vi "Elevator Controller.vi"(8 "error in":errorcluster) -> ()   [LabVIEW 2018]
doc: "This VI executes continuously carrying out the current operation and responding to updates or new operations. It will often contain the timing or control code that is difficult to place directly in TeleOp. This VI generally opens all sensors and motors and isolates the rest of the robot code from knowing how the operations are carried out."
uses:
  <vilib>/Rock Robotics/WPI/Framework/Completion Status.ctl
  Elevator Setpoints.ctl
  Elevator Operations.ctl
  <vilib>/Rock Robotics/WPI/SafetyOutput/WPI_SafetyOutputConfigMenu.ctl
  <vilib>/Rock Robotics/WPI/Utilities/WPI_GetSetVariantRefNum.vi
  <vilib>/Rock Robotics/Network Tables/NT Write Boolean.vi
panel:
  in  "Interactive Values":T1
  out "Current\nCmd":string
  in  "Buttons":cluster{"Execute Cmd":bool, "Abort Cmd":bool}
  out "Command Timing":cluster{"Start Time (ms)":u32, "Iterations":i32}
  out "Status":T3
  # "Tip: It may be helpful to observe inputs and sensor values.\nYou may also want to display tuning or debugging controls."
  # "Interactive Command: You may fill in the settings for a command\nand schedule it with the Execute button. You can observe and abort\nany command while fine tuning the code for the controller."
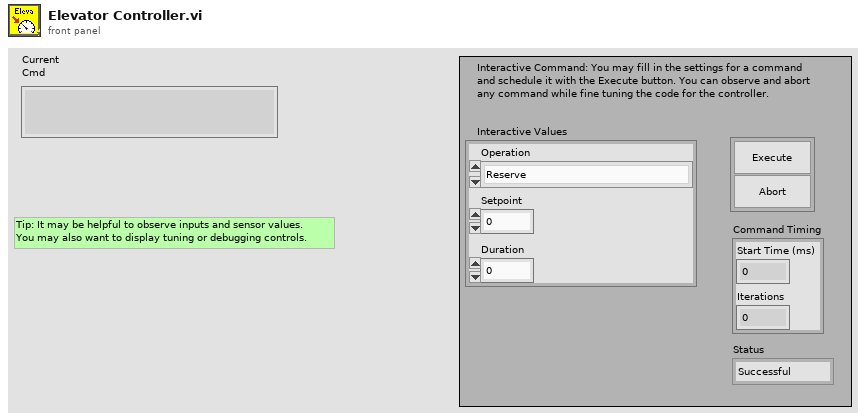
[diagram p1: front panel]
types:
  T1 = typedef "Elevator Setpoints.ctl" = cluster{"Operation":T2, "Setpoint":dbl, "Duration":dbl}
  T2 = typedef "Elevator Operations.ctl" = enum16{"Reserve", "Read Current", "Immediate"}
  T3 = typedef "Completion Status.ctl" = enum16{"Successful", "Aborted", "Incomplete"}
  T4 = typedef "WPI_SafetyOutputConfigMenu.ctl" = enum16{"Enable", "Disable"}
  T5 = typedef "WPI_RobotDriveDevRef.ctl" = cluster{"DevStatus":errorcluster, "Motors[]":T6[], "Square Inputs":bool, "Max Output":dbl}
  T6 = typedef "WPI_MotorControlDeviceRef.ctl" = cluster{"DeviceStatus":errorcluster, "Type":T7, "PWM":cluster{"PWM Channel":T8, "DeadBand":T9}, "CAN":cluster{"Device Number":u8, "SetOutput VI Ref":variant, "GetOutput VI Ref":variant, "Enable VI Ref":variant, "Disable VI Ref":variant, "Data":variant}, "Invert":bool, "DIO PWM":cluster{"PWM \"Enable\" Channel":T8, "DIOChannel":T10, "PWM Rate":dbl}}
  T7 = typedef "WPI_MotorControlType.ctl" = enum16{"PWM", "CAN", "DIO PWM"}
  T8 = typedef "FPGA_DIOPWMChannel.ctl" = enum8{"PWM 0", "PWM 1", "PWM 2", "PWM 3", "PWM 4", "PWM 5", "PWM 6", "PWM 7", "PWM 8", "PWM 9", "PWM MXP 0", "PWM MXP 1", "PWM MXP 2", "PWM MXP 3", "PWM MXP 4", "PWM MXP 5", "PWM MXP 6", "PWM MXP 7", "PWM MXP 8", "PWM MXP 9", "Invalid"}
  T9 = typedef "WPI_PWMDeadband.ctl" = cluster{"Name":string, "maxPositivePwm":i32, "minPositivePwm":i32, "centerPwm":i32, "maxNegativePwm":i32, "minNegativePwm":i32, "angularRange":u16}
  T10 = typedef "FPGA_DIOChannel.ctl" = enum8{"DIO 0", "DIO 1", "DIO 2", "DIO 3", "DIO 4", "DIO 5", "DIO 6", "DIO 7", "DIO 8", "DIO 9", "DIO MXP 0", "DIO MXP 1", "DIO MXP 2", "DIO MXP 3", "DIO MXP 4", "DIO MXP 5", "DIO MXP 6", "DIO MXP 7", "DIO MXP 8", "DIO MXP 9", "DIO MXP 10", "DIO MXP 11", "DIO MXP 12", "DIO MXP 13", "DIO MXP 14", "DIO MXP 15", "SPI Port CS1", "SPI Port CS2", "SPI Port CS3", "SPI Port MISO", "SPI Port MOSI", "Invalid"}
  T11 = typedef "Command Status Info.ctl" = cluster{"Name":string, "Status":T3, "notifier out":T12}
  T12 = typedef "Completion Notifier.ctl" = refnum<notifier>
  T13 = cluster{"Current Command":T1, "Command Timing":cluster{"Start Time (ms)":u32, "Iterations":i32}, "Command Arguments":cluster{"Command Info":T11, "Description":string, "Default Command":T1, "queue out":refnum<queue>, "Subsystem Name":string}}
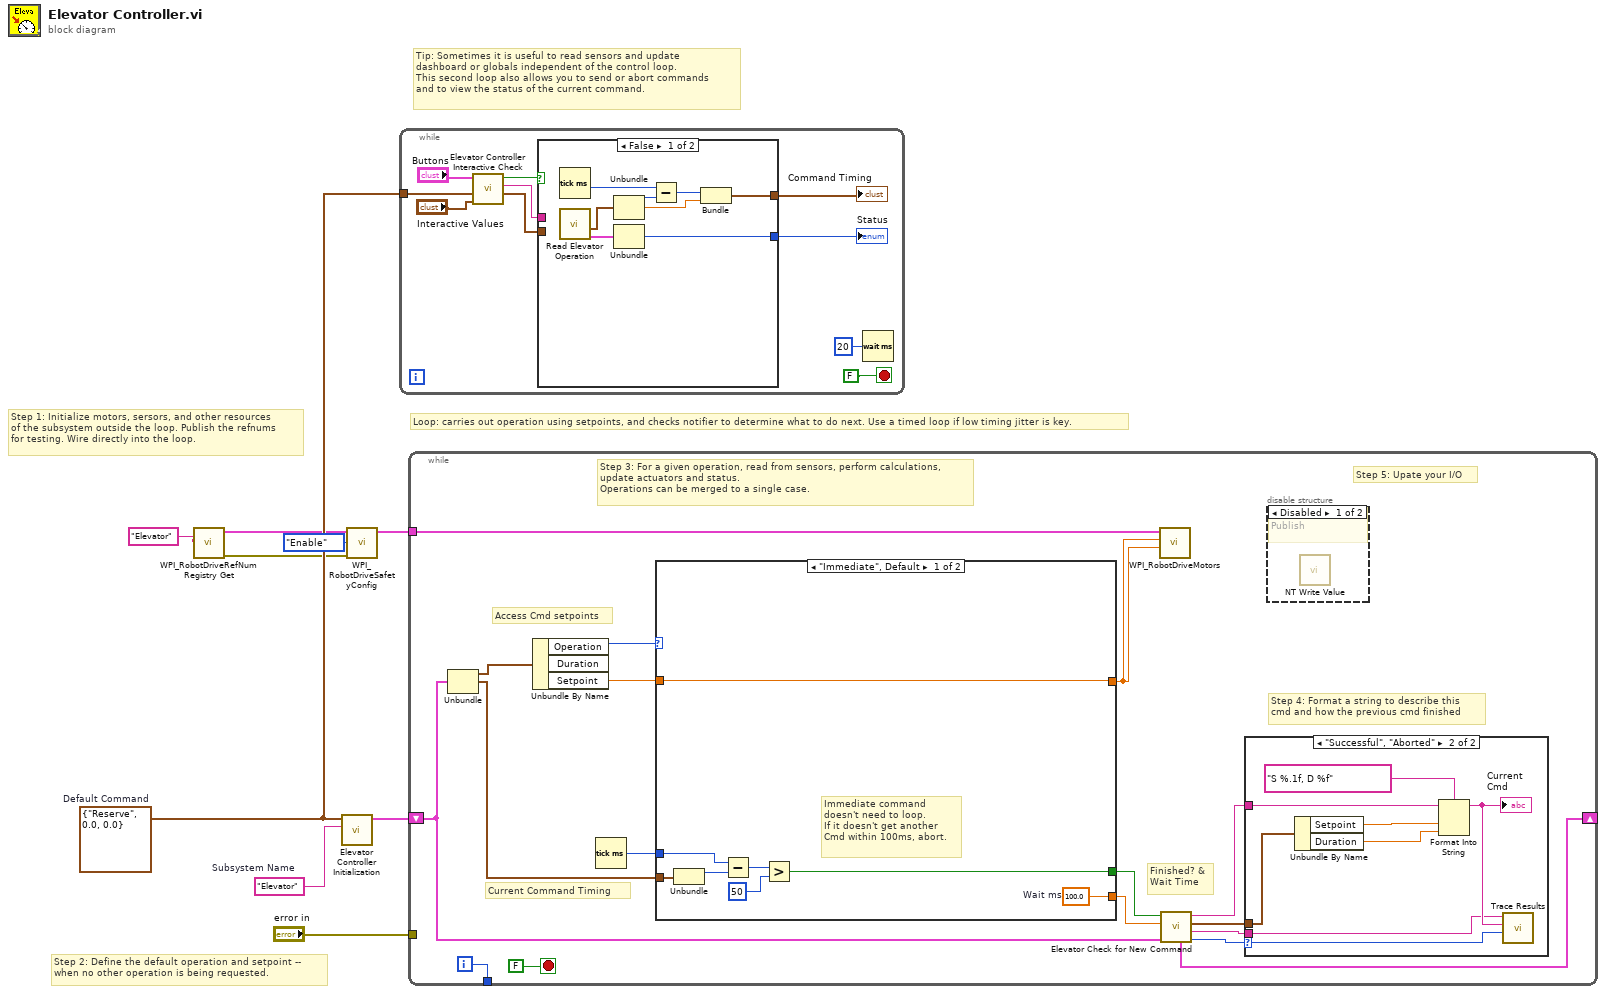
[diagram p0: block diagram]
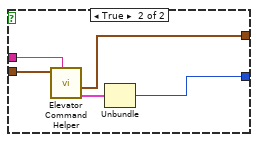
[diagram p2: hidden frame]
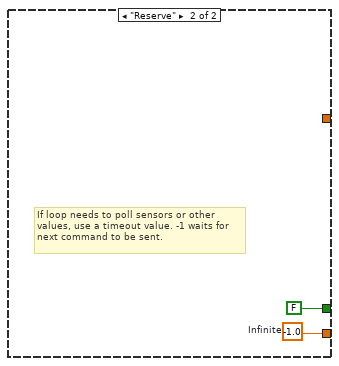
[diagram p5: hidden frame]
diagram:
  w6 = T1 {"Operation"=enum."Reserve", "Setpoint"=0.0, "Duration"=0.0}  # Default Command
  w7 = "Elevator"  # Subsystem Name
  # "Tip: Sometimes it is useful to read sensors and update\ndashboard or globals independent of the control loop.\nThis second loop also allows you to send or abort commands\nand to view the status of the current command."
  # "Step 2: Define the default operation and setpoint --\nwhen no other operation is being requested."
  # "Step 1: Initialize motors, sersors, and other resources\nof the subsystem outside the loop. Publish the refnums\nfor testing. Wire directly into the loop."
  # "Loop: carries out operation using setpoints, and checks notifier to determine what to do next. Use a timed loop if low timing jitter is key."
  n1 = call <vilib>:"WPI_RobotDriveRefNum Registry Get.vi"("refnum name"="Elevator") -> ("error out"=w5:errorcluster, "RobotDriveDevRef"=w4:T5)  [unwired: 9 in]
  n2 = call "Elevator Controller Initialization.vi"("Subsystem Name"=w7, "Default Command"=w6) -> ("Current Command"=w8:T13)  [unwired: 9 in]
  n3 = call <vilib>:"WPI_RobotDriveSafetyConfig.vi"("error in (no error)"=w5, "mode"=WPI_SafetyOutputConfigMenu."Enable", "RobotDriveDevRef"=w4) -> ("RobotDriveDevRef"=w1:T5)  [unwired: 7 in, 1 out]
  n4 = while {
    tunnel: w6 -> [w16]
    stop <- FALSE stop-if-true
    n5 = call "Elevator Controller Interactive Check.vi"("Interactive Command in"="Interactive Values", "Default Command"=w16, "Buttons"="Buttons") -> ("Interactive Command out"=w13:T1, "Trace String"=w14:string, "Schedule"=w15:bool)  [unwired: 6 in]
    n6 = case shown="False" w15 {
      tunnel: [w27 w32] -> w12
      tunnel: w13 -> [_ w30]
      tunnel: [w23 w28] -> w11
      tunnel: w14 -> [_ w31]
      frame False {
        n7 = Tick Count (ms)() -> (millisecond timer value=w22:u32)
        n8 = call "Read Elevator Operation.vi"() -> ("Command Info"=w20:T11, "SubSystem Data"=w21:T1)  [unwired: 9 in, 1 out]
        n9 = Unbundle(w21) -> ("Operation"=w26:T2, "Setpoint"=w24:dbl)  [unwired: 1 out]
        n10 = Unbundle(w20) -> ("Status"=w27:T3)  [unwired: 2 out]
        n11 = Subtract(x=w22, y=w26) -> (x-y=w25:u32)
        n12 = Bundle(w25, "Setpoint"=w24) -> (w23:cluster{u32, "Setpoint":dbl})  [unwired: 1 in]
      }
      frame True {
        n13 = call "Elevator Command Helper.vi"("Description"=w31, "SubSystem Data"=w30) -> ("Command Info Out"=w29:T11, "Command Timing"=w28:cluster{"Start Time (ms)":u32, "Iterations":i32})  [unwired: 7 in, 1 out]
        n14 = Unbundle(w29) -> ("Status"=w32:T3)  [unwired: 2 out]
      }
    }
    "Status" <- w12
    "Command Timing" <- w11
    n15 = Wait (ms)(milliseconds to wait=u32 20) -> ()  [unwired: 1 out]
  }
  n16 = while {
    shift-right: [w43] -> _
    shift-left: w8 -> [w36]
    tunnel: [w48] -> _
    tunnel: "error in" -> [_]
    tunnel: w1 -> [w34]
    i -> [w48]
    stop <- FALSE stop-if-true
    # "Step 5: Upate your I/O"
    # "Step 4: Format a string to describe this\ncmd and how the previous cmd finished"
    # "Current Command Timing"
    # "Access Cmd setpoints"
    # "Finished? &\nWait Time"
    # "Step 3: For a given operation, read from sensors, perform calculations,\nupdate actuators and status.\nOperations can be merged to a single case."
    n17 = Unbundle(w36) -> ("Current Command"=w47:T1, "Command Timing"=w44:cluster{"Start Time (ms)":u32, "Iterations":i32})  [unwired: 1 out]
    n18 = Unbundle By Name(w47) -> ("Operation"=w46:T2, "Setpoint"=w35:dbl)  [unwired: 1 out]
    n19 = Tick Count (ms)() -> (millisecond timer value=w45:u32)
    n20 = case shown="\"Immediate\", Default" w46 {
      tunnel: [w65 w67] -> w41
      tunnel: [w59 FALSE ("ignore previous (F)")] -> w42
      tunnel: w44 -> [w61 _]
      tunnel: w45 -> [w60 _]
      tunnel: [w58 _] -> w33
      tunnel: w35 -> [w58 _]
      frame "Immediate", Default {
        w65 = 100.0  # Wait ms
        # "Immediate command\ndoesn't need to loop.\nIf it doesn't get another\nCmd within 100ms, abort."
        n21 = Unbundle(w61) -> ("Start Time (ms)"=w64:u32)  [unwired: 1 out]
        n22 = Subtract(x=w60, y=w64) -> (x-y=w63:u32)
        n23 = Greater?(x=w63, y=u8 50 ("Left Motor")) -> (0:w59:bool)
      }
      frame "Reserve" {
        w67 = -1.0  # Infinite
        # "If loop needs to poll sensors or other\nvalues, use a timeout value. -1 waits for\nnext command to be sent."
      }
    }
    n24 = call <vilib>:"WPI_RobotDriveMotors.vi"("RightSpeed"=w33, "LeftSpeed"=w33, "RobotDriveDevRef"=w34) -> ()  [unwired: 6 in, 3 out]
    n25 = call "Elevator Check for New Command.vi"("Current Command"=w36, "Wait time (ms)"=w41, "Finished?"=w42) -> ("Completion"=w37:T3, "Subsystem Name"=w38:string, "Current Command"=w39:T1, "Initial Trace String"=w40:string, "NextCommand"=w43:T13)  [unwired: 4 in]
    n26 = case shown="\"Successful\", \"Aborted\"" w37 {
      selector: w37 -> [_ w57]
      tunnel: w40 -> [_ w53]
      tunnel: w39 -> [_ w54]
      tunnel: w38 -> [_ w50]
      frame "Incomplete", Default {
        # "Continuing current command"
      }
      frame "Successful", "Aborted" {
        # "Report and setup for next command"
        n27 = Unbundle By Name(w54) -> ("Setpoint"=w56:dbl, "Duration"=w51:dbl)
        n28 = Format Into String(format string="S %.1f, D %f", initial string=w53, w56, w51) -> (resulting string=w52:string)  [unwired: 1 in, 1 out]
        "Current\nCmd" <- w52
        n29 = call <vilib>:"Trace Results.vi"("Status of previous command"=w57, "Description"=w52, "Subsystem"=w50) -> ()  [unwired: 9 in]
      }
    }
    n30 = disable-structure shown="Disabled" {
      frame Disabled {
        # "Publish"
        n31 = call-poly <vilib>:"NT Write Value.vi"() -> ()  [unwired: 11 in, 1 out]
      }
      frame Enabled {
      }
    }
  }
